vi "Robot Global Data.vi"() -> ()   [LabVIEW 2011]
doc: "This global VI can contain as many global variables as you need. Place a control on the panel, give it a good name. To read or write to it from a VI, drag the icon to the diagram of that VI. You can also drag from the project. Click on the node to change which global you access. You shouldn't have multiple locations writing to a global or it will cause a race-condition."
uses:
  <vilib>/Rock Robotics/WPI/Camera/WPI_CameraImageSize.ctl
panel:
  out "IR Sensors":T1
  out "gyro":dbl
  out "Mast encoder":dbl
  out "Drive train":dbl
  out "IR bottom":bool
  out "Encoder Distance":dbl
  out "Arm up":bool
  out "Arm down":bool
  in  "LED toggle rate (ms)":u32
  in  "image size":T2=enum."320x240"
  in  "Enable Vision":bool
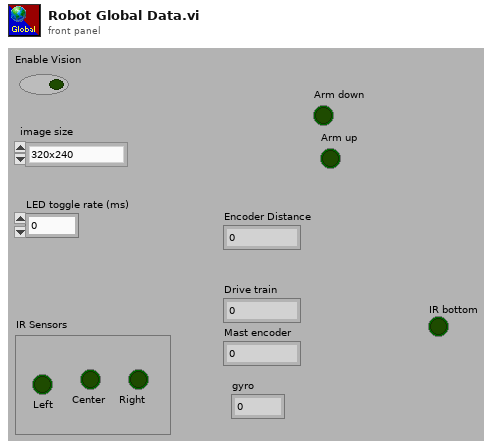
[diagram p1: front panel]
types:
  T1 = cluster{"Left":bool, "Center":bool, "Right":bool}
  T2 = typedef "WPI_CameraImageSize.ctl" = enum16{"640x480", "320x240", "160x120"}
diagram:
